vi "axis.vi"() -> (3 "reference out":refnum<vi>)   [LabVIEW 2011]
uses:
  <vilib>/picture/3D Picture Control/NI_3D Picture Control.lvlib
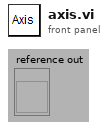
[diagram p1: front panel]
types:
  T1 = cluster{"Red":sgl, "Green":sgl, "Blue":sgl, "Alpha":sgl}
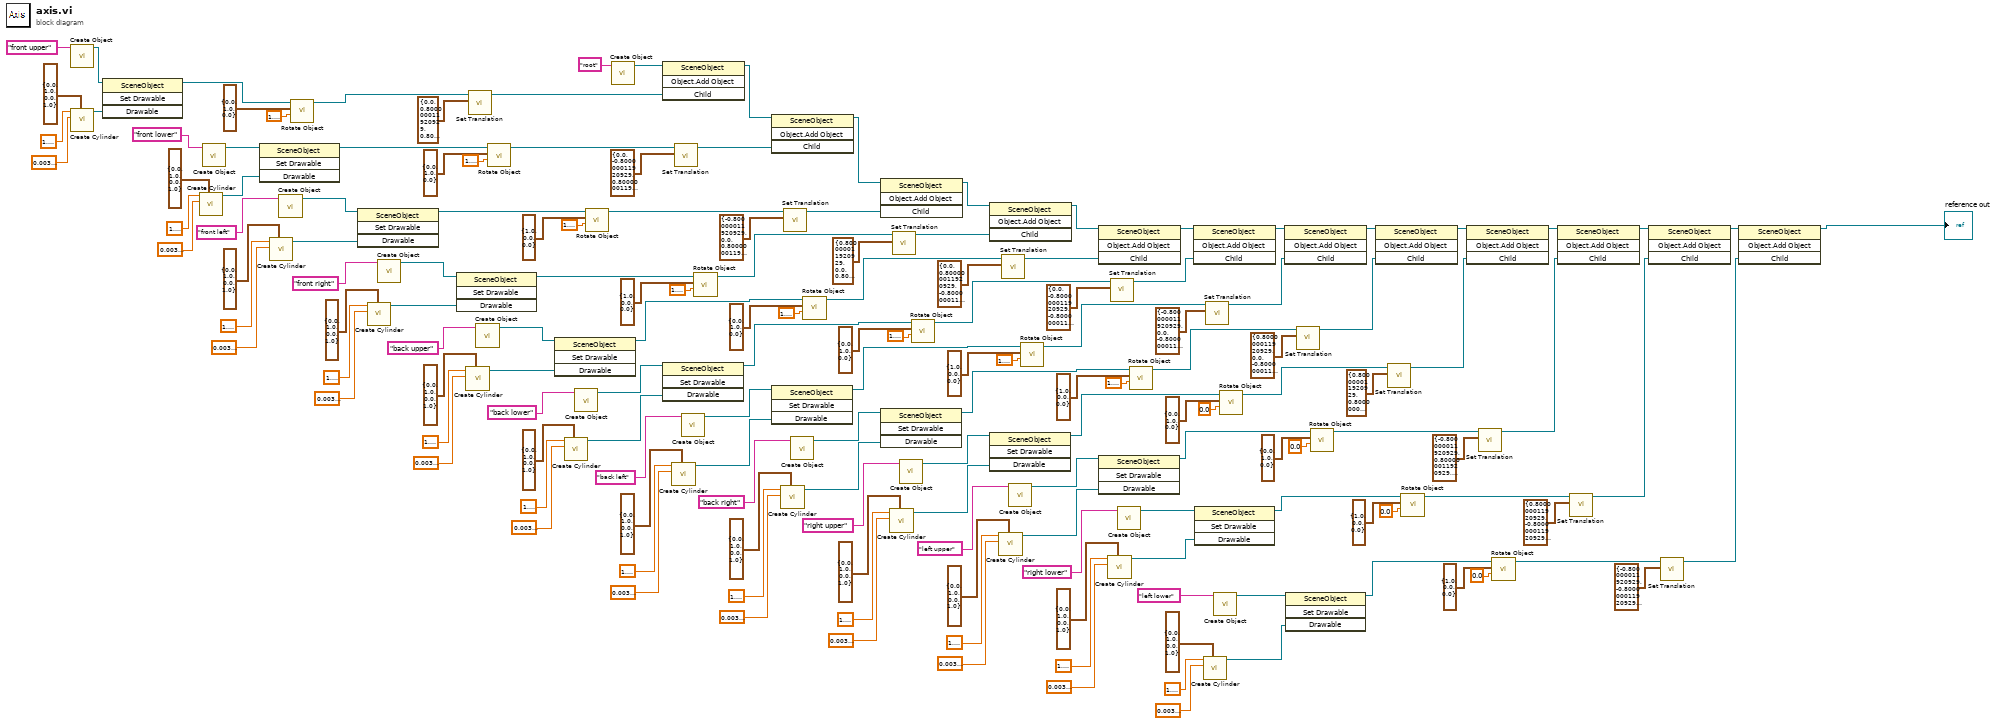
[diagram p0: block diagram]
diagram:
  n1 = call <vilib>:"Create Object.vi"("Name"="front upper") -> ("Scene:New Object"=w156:refnum<vi>)  [unwired: 9 in, 1 out]
  n2 = call <vilib>:"Create Cylinder.vi"("Color"=T1 {"Red"=0.0, "Green"=1.0, "Blue"=0.0, "Alpha"=1.0}, "Radius"=sgl 0.003, "Height"=sgl 1.6) -> ("New Cylinder Refnum"=w155:refnum<vi>)  [unwired: 7 in, 1 out]
  n3 = invoke class="SceneObject" method="Set Drawable"(reference=w156, "Drawable"=w155) -> (reference out=w154:refnum<vi>)  [unwired: 2 in, 3 out]
  n4 = call <vilib>:"Create Cylinder.vi"("Color"=T1 {"Red"=0.0, "Green"=1.0, "Blue"=0.0, "Alpha"=1.0}, "Radius"=sgl 0.003, "Height"=sgl 1.6) -> ("New Cylinder Refnum"=w142:refnum<vi>)  [unwired: 7 in, 1 out]
  n5 = call <vilib>:"Create Object.vi"("Name"="front lower") -> ("Scene:New Object"=w143:refnum<vi>)  [unwired: 9 in, 1 out]
  n6 = invoke class="SceneObject" method="Set Drawable"(reference=w143, "Drawable"=w142) -> (reference out=w141:refnum<vi>)  [unwired: 2 in, 3 out]
  n7 = call <vilib>:"Create Cylinder.vi"("Color"=T1 {"Red"=0.0, "Green"=1.0, "Blue"=0.0, "Alpha"=1.0}, "Radius"=sgl 0.003, "Height"=sgl 1.6) -> ("New Cylinder Refnum"=w128:refnum<vi>)  [unwired: 7 in, 1 out]
  n8 = call <vilib>:"Create Object.vi"("Name"="front left") -> ("Scene:New Object"=w129:refnum<vi>)  [unwired: 9 in, 1 out]
  n9 = call <vilib>:"Rotate Object.vi"("Angle"=1.5707963267948966, "Axis"=cluster{"X":sgl, "Y":sgl, "Z":sgl} {"X"=0.0, "Y"=1.0, "Z"=0.0}, "Scene.Object In"=w154) -> ("Scene.Object Out"=w150:refnum<vi>)  [unwired: 7 in, 1 out]
  n10 = invoke class="SceneObject" method="Set Drawable"(reference=w129, "Drawable"=w128) -> (reference out=w127:refnum<vi>)  [unwired: 2 in, 3 out]
  n11 = call <vilib>:"Create Cylinder.vi"("Color"=T1 {"Red"=0.0, "Green"=1.0, "Blue"=0.0, "Alpha"=1.0}, "Radius"=sgl 0.003, "Height"=sgl 1.6) -> ("New Cylinder Refnum"=w119:refnum<vi>)  [unwired: 7 in, 1 out]
  n12 = call <vilib>:"Create Object.vi"("Name"="front right") -> ("Scene:New Object"=w120:refnum<vi>)  [unwired: 9 in, 1 out]
  n13 = invoke class="SceneObject" method="Set Drawable"(reference=w120, "Drawable"=w119) -> (reference out=w118:refnum<vi>)  [unwired: 2 in, 3 out]
  n14 = call <vilib>:"Create Cylinder.vi"("Color"=T1 {"Red"=0.0, "Green"=1.0, "Blue"=0.0, "Alpha"=1.0}, "Radius"=sgl 0.003, "Height"=sgl 1.6) -> ("New Cylinder Refnum"=w104:refnum<vi>)  [unwired: 7 in, 1 out]
  n15 = call <vilib>:"Set Translation.vi"("Translation"=cluster{"X":sgl, "Y":sgl, "Z":sgl} {"X"=0.0, "Y"=0.8, "Z"=0.8}, "Scene Object"=w150) -> ("Translated Object"=w148:refnum<vi>)  [unwired: 8 in, 1 out]
  n16 = call <vilib>:"Create Object.vi"("Name"="back upper") -> ("Scene:New Object"=w105:refnum<vi>)  [unwired: 9 in, 1 out]
  n17 = call <vilib>:"Rotate Object.vi"("Angle"=1.5707963267948966, "Axis"=cluster{"X":sgl, "Y":sgl, "Z":sgl} {"X"=0.0, "Y"=1.0, "Z"=0.0}, "Scene.Object In"=w141) -> ("Scene.Object Out"=w137:refnum<vi>)  [unwired: 7 in, 1 out]
  n18 = invoke class="SceneObject" method="Set Drawable"(reference=w105, "Drawable"=w104) -> (reference out=w103:refnum<vi>)  [unwired: 2 in, 3 out]
  n19 = call <vilib>:"Create Cylinder.vi"("Color"=T1 {"Red"=0.0, "Green"=1.0, "Blue"=0.0, "Alpha"=1.0}, "Radius"=sgl 0.003, "Height"=sgl 1.6) -> ("New Cylinder Refnum"=w92:refnum<vi>)  [unwired: 7 in, 1 out]
  n20 = call <vilib>:"Create Object.vi"("Name"="back lower") -> ("Scene:New Object"=w93:refnum<vi>)  [unwired: 9 in, 1 out]
  n21 = call <vilib>:"Rotate Object.vi"("Angle"=1.5707963267948966, "Axis"=cluster{"X":sgl, "Y":sgl, "Z":sgl} {"X"=1.0, "Y"=0.0, "Z"=0.0}, "Scene.Object In"=w127) -> ("Scene.Object Out"=w113:refnum<vi>)  [unwired: 7 in, 1 out]
  n22 = call <vilib>:"Create Object.vi"("Name"="root") -> ("Scene:New Object"=w2:refnum<vi>)  [unwired: 9 in, 1 out]
  n23 = invoke class="SceneObject" method="Object.Add Object"(reference=w2, "Child"=w148) -> (reference out=w146:refnum<vi>)  [unwired: 2 in, 3 out]
  n24 = invoke class="SceneObject" method="Set Drawable"(reference=w93, "Drawable"=w92) -> (reference out=w91:refnum<vi>)  [unwired: 2 in, 3 out]
  n25 = call <vilib>:"Create Cylinder.vi"("Color"=T1 {"Red"=0.0, "Green"=1.0, "Blue"=0.0, "Alpha"=1.0}, "Radius"=sgl 0.003, "Height"=sgl 1.6) -> ("New Cylinder Refnum"=w78:refnum<vi>)  [unwired: 7 in, 1 out]
  n26 = call <vilib>:"Set Translation.vi"("Translation"=cluster{"X":sgl, "Y":sgl, "Z":sgl} {"X"=0.0, "Y"=-0.8, "Z"=0.8}, "Scene Object"=w137) -> ("Translated Object"=w134:refnum<vi>)  [unwired: 8 in, 1 out]
  n27 = call <vilib>:"Create Object.vi"("Name"="back left") -> ("Scene:New Object"=w79:refnum<vi>)  [unwired: 9 in, 1 out]
  n28 = call <vilib>:"Rotate Object.vi"("Angle"=1.5707963267948966, "Axis"=cluster{"X":sgl, "Y":sgl, "Z":sgl} {"X"=1.0, "Y"=0.0, "Z"=0.0}, "Scene.Object In"=w118) -> ("Scene.Object Out"=w112:refnum<vi>)  [unwired: 7 in, 1 out]
  n29 = invoke class="SceneObject" method="Object.Add Object"(reference=w146, "Child"=w134) -> (reference out=w133:refnum<vi>)  [unwired: 2 in, 3 out]
  n30 = invoke class="SceneObject" method="Set Drawable"(reference=w79, "Drawable"=w78) -> (reference out=w77:refnum<vi>)  [unwired: 2 in, 3 out]
  n31 = call <vilib>:"Create Cylinder.vi"("Color"=T1 {"Red"=0.0, "Green"=1.0, "Blue"=0.0, "Alpha"=1.0}, "Radius"=sgl 0.003, "Height"=sgl 1.6) -> ("New Cylinder Refnum"=w71:refnum<vi>)  [unwired: 7 in, 1 out]
  n32 = call <vilib>:"Set Translation.vi"("Translation"=cluster{"X":sgl, "Y":sgl, "Z":sgl} {"X"=-0.8, "Y"=0.0, "Z"=0.8}, "Scene Object"=w113) -> ("Translated Object"=w111:refnum<vi>)  [unwired: 8 in, 1 out]
  n33 = call <vilib>:"Create Object.vi"("Name"="back right") -> ("Scene:New Object"=w72:refnum<vi>)  [unwired: 9 in, 1 out]
  n34 = call <vilib>:"Rotate Object.vi"("Angle"=1.5707963267948966, "Axis"=cluster{"X":sgl, "Y":sgl, "Z":sgl} {"X"=0.0, "Y"=1.0, "Z"=0.0}, "Scene.Object In"=w103) -> ("Scene.Object Out"=w99:refnum<vi>)  [unwired: 7 in, 1 out]
  n35 = invoke class="SceneObject" method="Object.Add Object"(reference=w133, "Child"=w111) -> (reference out=w132:refnum<vi>)  [unwired: 2 in, 3 out]
  n36 = invoke class="SceneObject" method="Set Drawable"(reference=w72, "Drawable"=w71) -> (reference out=w70:refnum<vi>)  [unwired: 2 in, 3 out]
  n37 = call <vilib>:"Create Cylinder.vi"("Color"=T1 {"Red"=0.0, "Green"=1.0, "Blue"=0.0, "Alpha"=1.0}, "Radius"=sgl 0.003, "Height"=sgl 1.6) -> ("New Cylinder Refnum"=w52:refnum<vi>)  [unwired: 7 in, 1 out]
  n38 = call <vilib>:"Set Translation.vi"("Translation"=cluster{"X":sgl, "Y":sgl, "Z":sgl} {"X"=0.8, "Y"=0.0, "Z"=0.8}, "Scene Object"=w112) -> ("Translated Object"=w110:refnum<vi>)  [unwired: 8 in, 1 out]
  n39 = call <vilib>:"Create Object.vi"("Name"="right upper") -> ("Scene:New Object"=w53:refnum<vi>)  [unwired: 9 in, 1 out]
  n40 = call <vilib>:"Rotate Object.vi"("Angle"=1.5707963267948966, "Axis"=cluster{"X":sgl, "Y":sgl, "Z":sgl} {"X"=0.0, "Y"=1.0, "Z"=0.0}, "Scene.Object In"=w91) -> ("Scene.Object Out"=w87:refnum<vi>)  [unwired: 7 in, 1 out]
  n41 = invoke class="SceneObject" method="Object.Add Object"(reference=w132, "Child"=w110) -> (reference out=w58:refnum<vi>)  [unwired: 2 in, 3 out]
  n42 = invoke class="SceneObject" method="Set Drawable"(reference=w53, "Drawable"=w52) -> (reference out=w51:refnum<vi>)  [unwired: 2 in, 3 out]
  n43 = call <vilib>:"Create Cylinder.vi"("Color"=T1 {"Red"=0.0, "Green"=1.0, "Blue"=0.0, "Alpha"=1.0}, "Radius"=sgl 0.003, "Height"=sgl 1.6) -> ("New Cylinder Refnum"=w42:refnum<vi>)  [unwired: 7 in, 1 out]
  n44 = call <vilib>:"Set Translation.vi"("Translation"=cluster{"X":sgl, "Y":sgl, "Z":sgl} {"X"=0.0, "Y"=0.8, "Z"=-0.8}, "Scene Object"=w99) -> ("Translated Object"=w59:refnum<vi>)  [unwired: 8 in, 1 out]
  n45 = call <vilib>:"Create Object.vi"("Name"="left upper") -> ("Scene:New Object"=w43:refnum<vi>)  [unwired: 9 in, 1 out]
  n46 = call <vilib>:"Rotate Object.vi"("Angle"=1.5707963267948966, "Axis"=cluster{"X":sgl, "Y":sgl, "Z":sgl} {"X"=1.0, "Y"=0.0, "Z"=0.0}, "Scene.Object In"=w77) -> ("Scene.Object Out"=w65:refnum<vi>)  [unwired: 7 in, 1 out]
  n47 = invoke class="SceneObject" method="Object.Add Object"(reference=w58, "Child"=w59) -> (reference out=w96:refnum<vi>)  [unwired: 2 in, 3 out]
  n48 = invoke class="SceneObject" method="Set Drawable"(reference=w43, "Drawable"=w42) -> (reference out=w41:refnum<vi>)  [unwired: 2 in, 3 out]
  n49 = call <vilib>:"Create Cylinder.vi"("Color"=T1 {"Red"=0.0, "Green"=1.0, "Blue"=0.0, "Alpha"=1.0}, "Radius"=sgl 0.003, "Height"=sgl 1.6) -> ("New Cylinder Refnum"=w30:refnum<vi>)  [unwired: 7 in, 1 out]
  n50 = call <vilib>:"Set Translation.vi"("Translation"=cluster{"X":sgl, "Y":sgl, "Z":sgl} {"X"=0.0, "Y"=-0.8, "Z"=-0.8}, "Scene Object"=w87) -> ("Translated Object"=w84:refnum<vi>)  [unwired: 8 in, 1 out]
  n51 = call <vilib>:"Create Object.vi"("Name"="right lower") -> ("Scene:New Object"=w9:refnum<vi>)  [unwired: 9 in, 1 out]
  n52 = call <vilib>:"Rotate Object.vi"("Angle"=1.5707963267948966, "Axis"=cluster{"X":sgl, "Y":sgl, "Z":sgl} {"X"=1.0, "Y"=0.0, "Z"=0.0}, "Scene.Object In"=w70) -> ("Scene.Object Out"=w64:refnum<vi>)  [unwired: 7 in, 1 out]
  n53 = invoke class="SceneObject" method="Object.Add Object"(reference=w96, "Child"=w84) -> (reference out=w83:refnum<vi>)  [unwired: 2 in, 3 out]
  n54 = invoke class="SceneObject" method="Set Drawable"(reference=w9, "Drawable"=w30) -> (reference out=w29:refnum<vi>)  [unwired: 2 in, 3 out]
  n55 = call <vilib>:"Create Cylinder.vi"("Color"=T1 {"Red"=0.0, "Green"=1.0, "Blue"=0.0, "Alpha"=1.0}, "Radius"=sgl 0.003, "Height"=sgl 1.6) -> ("New Cylinder Refnum"=w24:refnum<vi>)  [unwired: 7 in, 1 out]
  n56 = call <vilib>:"Set Translation.vi"("Translation"=cluster{"X":sgl, "Y":sgl, "Z":sgl} {"X"=-0.8, "Y"=0.0, "Z"=-0.8}, "Scene Object"=w65) -> ("Translated Object"=w63:refnum<vi>)  [unwired: 8 in, 1 out]
  n57 = call <vilib>:"Create Object.vi"("Name"="left lower") -> ("Scene:New Object"=w25:refnum<vi>)  [unwired: 9 in, 1 out]
  n58 = call <vilib>:"Rotate Object.vi"("Angle"=sgl 0.0, "Axis"=cluster{"X":sgl, "Y":sgl, "Z":sgl} {"X"=0.0, "Y"=1.0, "Z"=0.0}, "Scene.Object In"=w51) -> ("Scene.Object Out"=w48:refnum<vi>)  [unwired: 7 in, 1 out]
  n59 = invoke class="SceneObject" method="Object.Add Object"(reference=w83, "Child"=w63) -> (reference out=w82:refnum<vi>)  [unwired: 2 in, 3 out]
  n60 = invoke class="SceneObject" method="Set Drawable"(reference=w25, "Drawable"=w24) -> (reference out=w23:refnum<vi>)  [unwired: 2 in, 3 out]
  n61 = call <vilib>:"Set Translation.vi"("Translation"=cluster{"X":sgl, "Y":sgl, "Z":sgl} {"X"=0.8, "Y"=0.0, "Z"=-0.8}, "Scene Object"=w64) -> ("Translated Object"=w62:refnum<vi>)  [unwired: 8 in, 1 out]
  n62 = call <vilib>:"Rotate Object.vi"("Angle"=sgl 0.0, "Axis"=cluster{"X":sgl, "Y":sgl, "Z":sgl} {"X"=0.0, "Y"=1.0, "Z"=0.0}, "Scene.Object In"=w41) -> ("Scene.Object Out"=w38:refnum<vi>)  [unwired: 7 in, 1 out]
  n63 = invoke class="SceneObject" method="Object.Add Object"(reference=w82, "Child"=w62) -> (reference out=w10:refnum<vi>)  [unwired: 2 in, 3 out]
  n64 = call <vilib>:"Set Translation.vi"("Translation"=cluster{"X":sgl, "Y":sgl, "Z":sgl} {"X"=0.8, "Y"=0.8, "Z"=0.0}, "Scene Object"=w48) -> ("Translated Object"=w12:refnum<vi>)  [unwired: 8 in, 1 out]
  n65 = call <vilib>:"Rotate Object.vi"("Angle"=sgl 0.0, "Axis"=cluster{"X":sgl, "Y":sgl, "Z":sgl} {"X"=1.0, "Y"=0.0, "Z"=0.0}, "Scene.Object In"=w29) -> ("Scene.Object Out"=w19:refnum<vi>)  [unwired: 7 in, 1 out]
  n66 = invoke class="SceneObject" method="Object.Add Object"(reference=w10, "Child"=w12) -> (reference out=w11:refnum<vi>)  [unwired: 2 in, 3 out]
  n67 = call <vilib>:"Set Translation.vi"("Translation"=cluster{"X":sgl, "Y":sgl, "Z":sgl} {"X"=-0.8, "Y"=0.8, "Z"=0.0}, "Scene Object"=w38) -> ("Translated Object"=w35:refnum<vi>)  [unwired: 8 in, 1 out]
  n68 = call <vilib>:"Rotate Object.vi"("Angle"=sgl 0.0, "Axis"=cluster{"X":sgl, "Y":sgl, "Z":sgl} {"X"=1.0, "Y"=0.0, "Z"=0.0}, "Scene.Object In"=w23) -> ("Scene.Object Out"=w18:refnum<vi>)  [unwired: 7 in, 1 out]
  n69 = invoke class="SceneObject" method="Object.Add Object"(reference=w11, "Child"=w35) -> (reference out=w34:refnum<vi>)  [unwired: 2 in, 3 out]
  n70 = call <vilib>:"Set Translation.vi"("Translation"=cluster{"X":sgl, "Y":sgl, "Z":sgl} {"X"=0.8, "Y"=-0.8, "Z"=0.0}, "Scene Object"=w19) -> ("Translated Object"=w13:refnum<vi>)  [unwired: 8 in, 1 out]
  n71 = invoke class="SceneObject" method="Object.Add Object"(reference=w34, "Child"=w13) -> (reference out=w33:refnum<vi>)  [unwired: 2 in, 3 out]
  n72 = call <vilib>:"Set Translation.vi"("Translation"=cluster{"X":sgl, "Y":sgl, "Z":sgl} {"X"=-0.8, "Y"=-0.8, "Z"=0.0}, "Scene Object"=w18) -> ("Translated Object"=w17:refnum<vi>)  [unwired: 8 in, 1 out]
  n73 = invoke class="SceneObject" method="Object.Add Object"(reference=w33, "Child"=w17) -> (reference out=→"reference out":refnum<vi>)  [unwired: 2 in, 3 out]
